vi "NotifyIcon - Show BalloonTip.vi"(6 "display time (ms)":i32=5000, 7 "Icon (None)":i32(ring) items=["None", "Info", "Warning", "Error"], 8 "error in":errorcluster, 9 "Text":string, 10 "Title":string, 11 "NotifyIcon reference in":refnum<k24>) -> (0 "error out":errorcluster, 3 "NotifyIcon reference out":refnum<k24>)   [LabVIEW 2018]
doc: "Displays a Balloon Tip with the specified <b>Title</b>, <b>Text</b>, and <b>Icon</b> in the taskbar for the specified time period.\n\nInput <b>display time (ms)</b> is approximate (at best) and will be coerced depending on OS."
uses:
  System.Windows.Forms
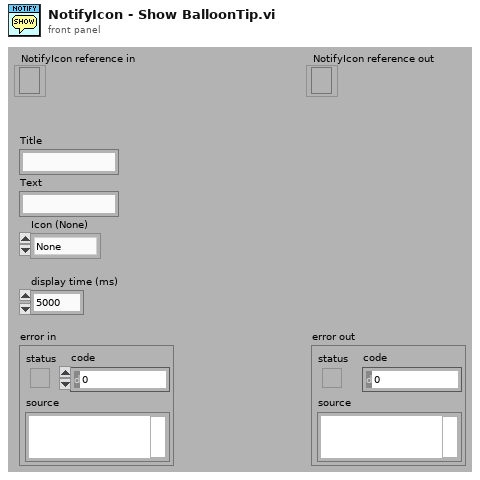
[diagram p1: front panel]
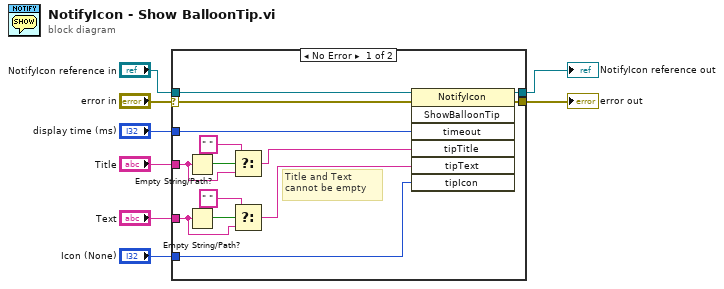
[diagram p0: block diagram]
diagram:
  n1 = case shown="No Error" "error in" {
    selector: "error in" -> [w9 w23]
    tunnel: "display time (ms)" -> [w22 _]
    tunnel: [w21 w24] -> w7
    tunnel: [w20 w23] -> w6
    tunnel: "NotifyIcon reference in" -> [w19 w24]
    tunnel: "Icon (None)" -> [w18 _]
    tunnel: "Title" -> [w16 _]
    tunnel: "Text" -> [w11 _]
    frame No Error {
      # "Title and Text\ncannot be empty"
      n2 = Empty String/Path?(string/path=w16) -> (empty?=w17:bool)
      n3 = Empty String/Path?(string/path=w11) -> (empty?=w12:bool)
      n4 = Select(t=" ", s=w17, f=w16) -> (s? t:f=w14:string)
      n5 = Select(t=" ", s=w12, f=w11) -> (s? t:f=w10:string)
      n6 = invoke class="NotifyIcon" method="ShowBalloonTip"(reference=w19, error in=w9, "timeout"=w22, "tipTitle"=w14, "tipText"=w10, "tipIcon"=w18) -> (reference out=w21:refnum<k24>, error out=w20:errorcluster)  [unwired: 1 in, 5 out]
    }
    frame Error {
    }
  }
  "NotifyIcon reference out" <- w7
  "error out" <- w6
